vi "OPCServer.vi"() -> ()   [LabVIEW 2026]
uses:
  <vilib>/OPCUA/controls/Data Type.ctl
  <vilib>/OPCUA/server/Create2.vi
  <vilib>/OPCUA/NI OPC UA Server.lvlib
  <vilib>/OPCUA/controls/NodeId.ctl
panel:
  out "Sensors":T1[](array[typedef])
  in  "Stop Button":bool
  out "server endpoint URL":string
  # "OPC Server"
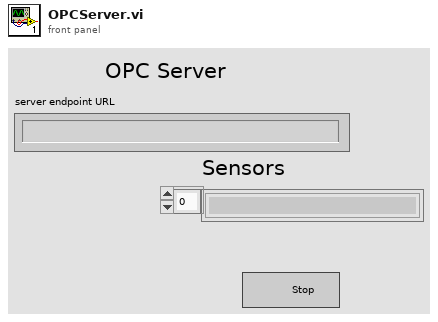
[diagram p1: front panel]
types:
  T1 = typedef "NodeId.ctl" = string
  T2 = typedef "OPC UA Server Refnum.ctl" = refnum<k21>
  T3 = typedef "Data Type.ctl" = u16
  T4 = cluster{"name":string, "data type":T3, "access level":u16, "description":string}
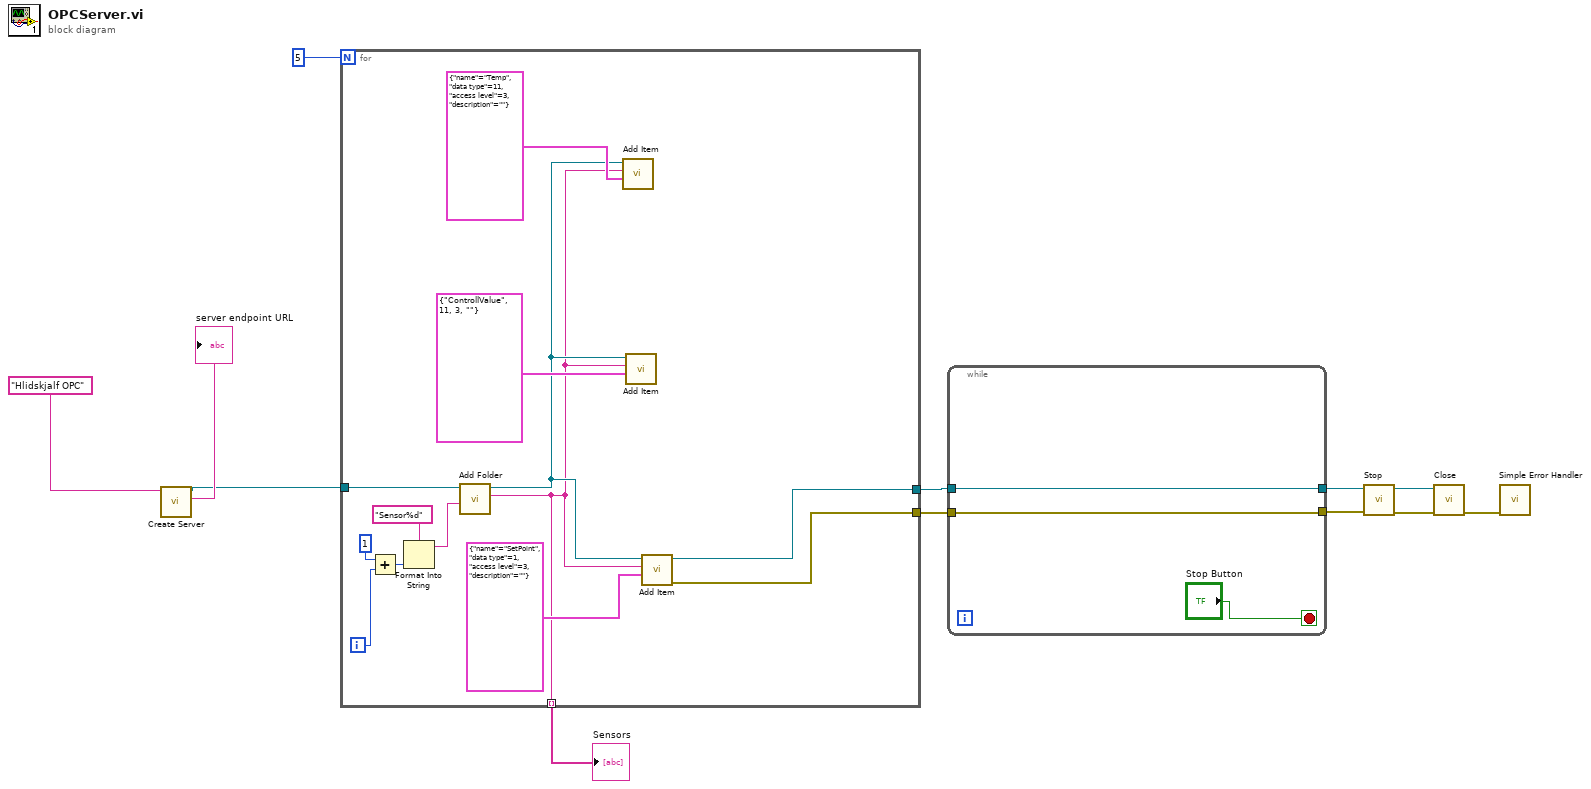
[diagram p0: block diagram]
diagram:
  n1 = call-poly <vilib>:"Create Server.vi"("OPC UA server name"="Hlidskjalf OPC") -> ("server endpoint URL"=→"server endpoint URL":string, "OPC UA server refnum out"=w5:T2)  [unwired: 8 in, 1 out]
  n2 = for {
    N: 5 -> [_]
    tunnel: w5 -> [w25]
    tunnel: [w16] -> w4
    tunnel: [w15] -> w3
    tunnel: [w13] -> w1 mode=indexing
    i -> [w22]
    n3 = Add(x=1, y=w22) -> (x+y=w23:i32)
    n4 = Format Into String(format string="Sensor%d", w23) -> (resulting string=w14:string)  [unwired: 2 in, 1 out]
    n5 = call <vilib>:"Add Folder.vi"("folder name"=w14, "OPC UA server refnum in"=w25) -> ("folder node ID"=w13:T1, "OPC UA server refnum out"=w17:T2)  [unwired: 6 in, 1 out]
    n6 = call <vilib>:"Add Item.vi"("item"=T4 {"name"="Temp", "data type"=11, "access level"=3, "description"=""}, "parent folder node ID"=w13, "OPC UA server refnum in"=w17) -> ()  [unwired: 4 in, 4 out]
    n7 = call <vilib>:"Add Item.vi"("item"=T4 {"name"="ControllValue", "data type"=11, "access level"=3, "description"=""}, "parent folder node ID"=w13, "OPC UA server refnum in"=w17) -> ()  [unwired: 4 in, 4 out]
    n8 = call <vilib>:"Add Item.vi"("item"=T4 {"name"="SetPoint", "data type"=1, "access level"=3, "description"=""}, "parent folder node ID"=w13, "OPC UA server refnum in"=w17) -> ("error out"=w15:errorcluster, "OPC UA server refnum out"=w16:T2)  [unwired: 4 in, 2 out]
  }
  "Sensors" <- w1
  n9 = while {
    tunnel: [w28] -> w7
    tunnel: w4 -> [w28]
    tunnel: [w27] -> w6
    tunnel: w3 -> [w27]
    stop <- "Stop Button" stop-if-true
  }
  n10 = call <vilib>:"Stop.vi"("error in (no error)"=w6, "OPC UA server refnum in"=w7) -> ("error out"=w10:errorcluster, "OPC UA server refnum out"=w9:T2)  [unwired: 8 in]
  n11 = call <vilib>:"Close.vi"("error in (no error)"=w10, "OPC UA server refnum in"=w9) -> ("error out"=w8:errorcluster)  [unwired: 9 in]
  n12 = call <vilib>:"Simple Error Handler.vi"("error in (no error)"=w8) -> ()  [unwired: 4 in, 5 out]
